vi "Get Nitrogen Level.vi"(8 "error in (no error)":errorcluster, 11 "Instrument.Cryostat in":refnum<class "Instrument.Cryostat.lvclass">) -> (0 "error out":errorcluster, 2 "LN2 Level (%)":dbl, 3 "Instrument.Cryostat out":refnum<class "Instrument.Cryostat.lvclass">)   [LabVIEW 2019, in "Instrument.Cryostat.lvclass"]
uses:
  Instrument.Cryostat.lvclass
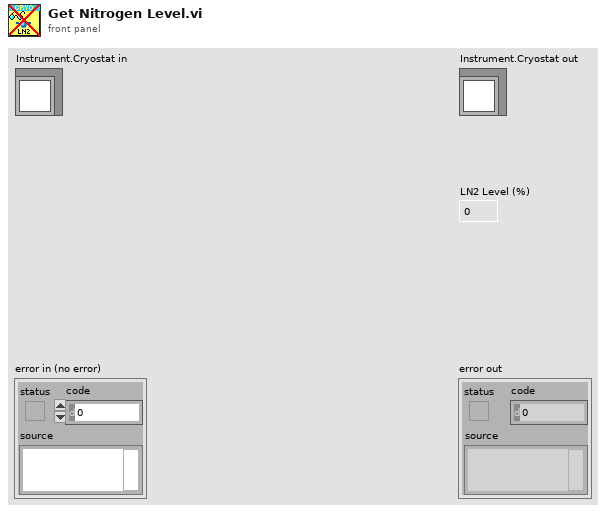
[diagram p1: front panel]
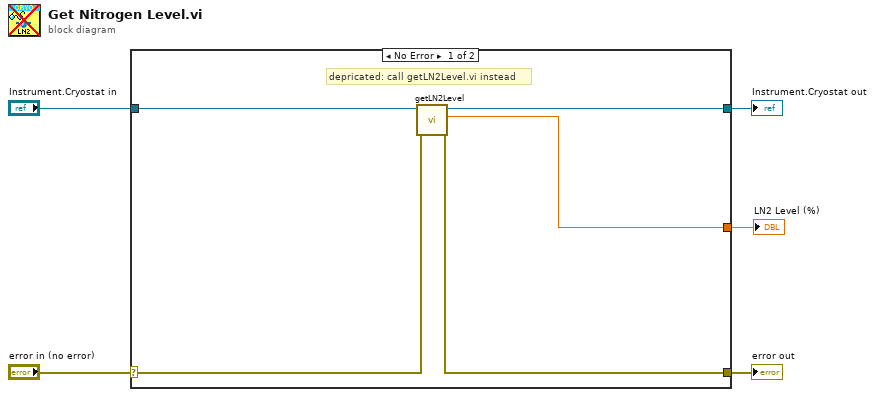
[diagram p0: block diagram]
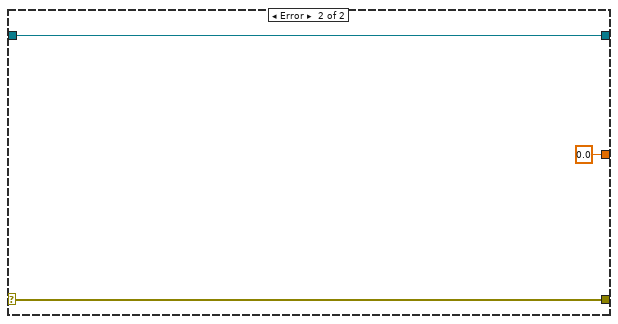
[diagram p2: hidden frame]
diagram:
  n1 = case shown="No Error" "error in (no error)" {
    selector: "error in (no error)" -> [w7 w13]
    tunnel: [w9 w13] -> w4
    tunnel: [w10 w12] -> w2
    tunnel: "Instrument.Cryostat in" -> [w8 w12]
    tunnel: [w6 0.0 ("LN2 Level (%)")] -> w1
    frame No Error {
      # "depricated: call getLN2Level.vi instead"
      n2 = call-dynamic "getLN2Level.vi"("error in (no error)"=w7, "Instrument.Cryostat in"=w8) -> ("error out"=w9:errorcluster, "LN2 Level (%)"=w6:dbl, "Instrument.Cryostat out"=w10:refnum<class "Instrument.Cryostat.lvclass">)  [unwired: 7 in]
    }
    frame Error {
    }
  }
  "error out" <- w4
  "Instrument.Cryostat out" <- w2
  "LN2 Level (%)" <- w1
